vi "Ini key read (Boolean).vi"(7 "Section":string, 8 "error in (no error)":errorcluster, 10 "Parameter names & setup":T2, 11 "Ini file refnum in":T1) -> (0 "error out":errorcluster, 2 "Value read/used":bool[](array[boolean]), 3 "Ini file refnum out":T1)   [LabVIEW 2013]
uses:
  Typedefs/Ini file interface (Boolean).ctl
  <vilib>/Utility/config.llb/Config Data RefNum.ctl
  <vilib>/Utility/config.llb/Read Key (Boolean).vi
  <vilib>/Utility/config.llb/Write Key (Boolean).vi
  <vilib>/Utility/config.llb/NI_LVConfig.lvlib
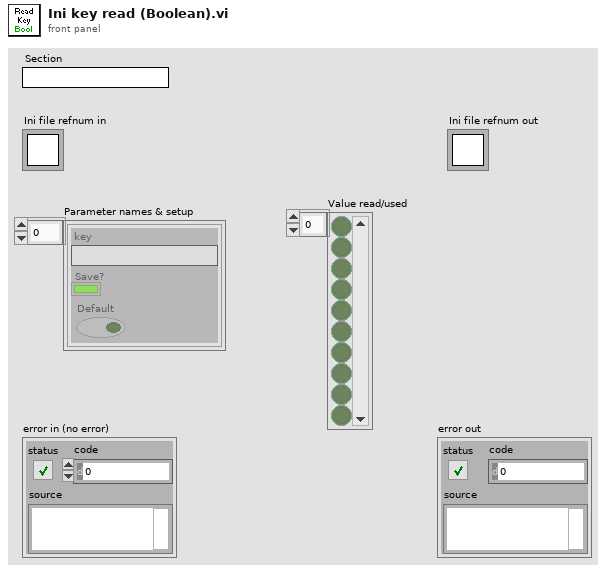
[diagram p1: front panel]
types:
  T1 = typedef "NI_LVConfig.lvlib/Config Data RefNum.ctl" = refnum<k1>
  T2 = typedef "Ini file interface (Boolean).ctl" = cluster{"key":string, "Save?":bool, "Default":bool}[]
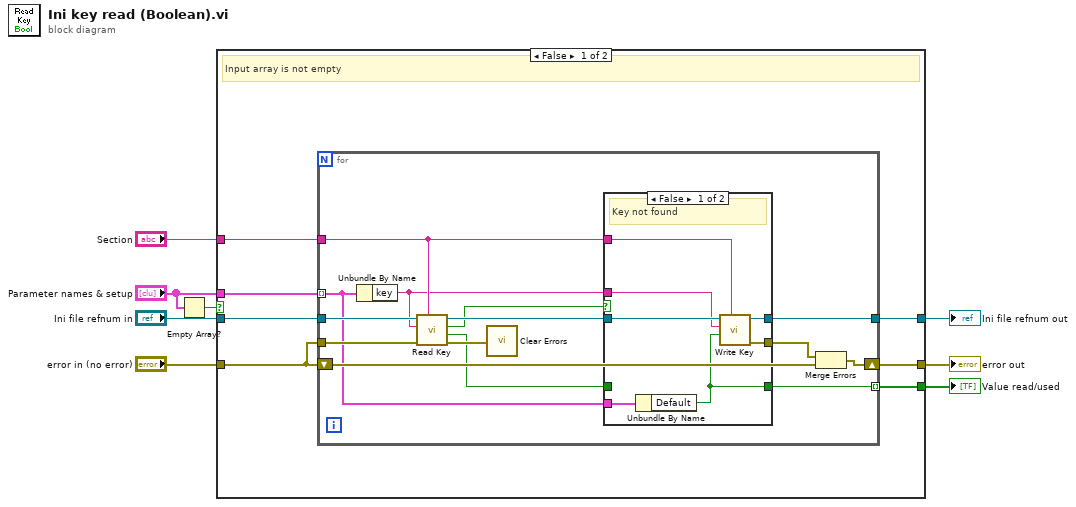
[diagram p0: block diagram]
diagram:
  n1 = Empty Array?(array="Parameter names & setup") -> (empty?=w1:bool)
  n2 = case shown="False" w1 {
    tunnel: "Section" -> [w9 _]
    tunnel: "Parameter names & setup" -> [w15 _]
    tunnel: [w14 _] -> w7
    tunnel: "error in (no error)" -> [w13 w39]
    tunnel: [w12 w39] -> w5
    tunnel: [w11 w40] -> w4
    tunnel: "Ini file refnum in" -> [w10 w40]
    frame False {
      # "Input array is not empty"
      n3 = for {
        tunnel: w9 -> [w18]
        tunnel: w10 -> [w29]
        tunnel: w13 -> [w28]
        tunnel: [w23] -> w11
        shift-right: [w27] -> w12
        shift-left: w13 -> [w26]
        tunnel: w15 -> [w19] mode=indexing
        tunnel: [w20] -> w14 mode=indexing
        n4 = Unbundle By Name(w19) -> ("key"=w17:string)
        n5 = call-poly <vilib>:"Read Key.vi"("section"=w18, "error in (no error)"=w28, "key"=w17, "refnum"=w29) -> ("error out"=w25:errorcluster, "value"=w21:bool, "found?"=w16:bool, "refnum out"=w24:T1)  [unwired: 4 in]
        n6 = call <vilib>:"Clear Errors.vi"("error in (no error)"=w25) -> ()  [unwired: 6 in, 1 out]
        n7 = case shown="False" w16 {
          tunnel: w24 -> [w36 w38]
          tunnel: [w35 w38] -> w23
          tunnel: [w34 _] -> w22
          tunnel: w18 -> [w33 _]
          tunnel: w17 -> [w32 _]
          tunnel: w21 -> [_ w37]
          tunnel: [w30 w37] -> w20
          tunnel: w19 -> [w31 _]
          frame False {
            # "Key not found"
            n8 = Unbundle By Name(w31) -> ("Default"=w30:bool)
            n9 = call-poly <vilib>:"Write Key.vi"("section"=w33, "value"=w30, "key"=w32, "refnum"=w36) -> ("error out"=w34:errorcluster, "refnum out"=w35:T1)  [unwired: 5 in, 1 out]
          }
          frame True {
            # "Key found"
          }
        }
        n10 = Merge Errors(w22, w26) -> (w27:errorcluster)
      }
    }
    frame True {
      # "Input array is empty"
    }
  }
  "Value read/used" <- w7
  "error out" <- w5
  "Ini file refnum out" <- w4
